vi "RSZVB Get Pulse Train Segments.vi"(8 "error in (no error)":errorcluster {"code" format="%.0x"}, 10 "Channel (1)":i32=1, 11 "VISA session":refnum<visa-resource-name>) -> (0 "error out":errorcluster {"code" format="%.0x"}, 1 "Pulse Train Active":i32[](array[numeric]), 3 "dup VISA session":refnum<visa-resource-name>, 4 "Start Time":dbl[](array[numeric]) format="%^.3e", 5 "Stop Time":dbl[](array[numeric]) format="%^.3e")   [LabVIEW 2011]
doc: "This VI returns the pulse train segments. Each segment consists of a single pulse of definite width and position which may be active or inactive.\n\nNote(s):\n\n(1) This VI is available only with option R&S ZVA-K27.\n\nRemote-control command(s):\n[SENSe<Ch>:]PULSe:GENerator<gen_no>:TRAin:DATA?"
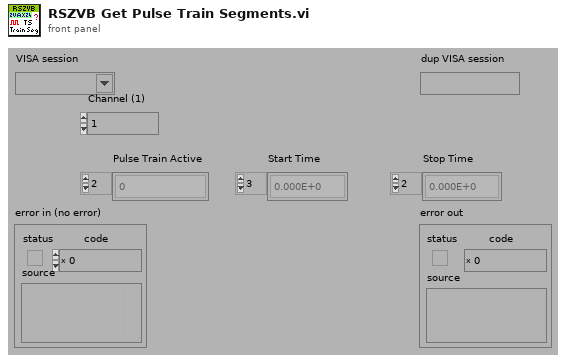
[diagram p1: front panel]
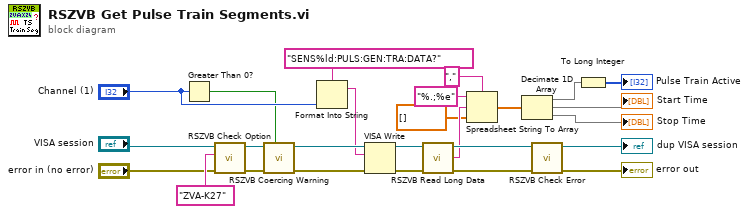
[diagram p0: block diagram]
diagram:
  n1 = Greater Than 0?(x="Channel (1)") -> (x > 0?=w16:bool)
  n2 = call "RSZVB Check Option.vi"("error in (no error)"="error in (no error)", "Options"="ZVA-K27", "VISA session"="VISA session") -> ("error out"=w22:errorcluster, "dup VISA session"=w21:refnum<visa-resource-name>)  [unwired: 7 in]
  n3 = call "RSZVB Coercing Warning.vi"("In Range?"=w16, "error in (no error)"=w22, "VISA session"=w21) -> ("error out"=w25:errorcluster, "dup VISA session"=w26:refnum<visa-resource-name>)  [unwired: 7 in]
  n4 = Format Into String(format string="SENS%ld:PULS:GEN:TRA:DATA?", "Channel (1)") -> (resulting string=w24:string)  [unwired: 2 in, 1 out]
  n5 = VISA Write(VISA resource name=w26, write buffer=w24, error in (no error)=w25) -> (VISA resource name out=w15:refnum<visa-resource-name>, error out=w14:errorcluster)  [unwired: 1 out]
  n6 = call "RSZVB Read Long Data.vi"("error in (no error)"=w14, "VISA resource name"=w15) -> ("error out"=w13:errorcluster, "Data"=w10:string, "VISA resource name out"=w12:refnum<visa-resource-name>)  [unwired: 7 in]
  n7 = Spreadsheet String To Array(delimiter (Tab)=",", format string="%.;%e", spreadsheet string=w10, array type (2D Dbl)=dbl[] [] ("Stop Time")) -> (array=w8:dbl[])
  n8 = Decimate 1D Array(w8) -> (w6:dbl[], →"Start Time":dbl[], →"Stop Time":dbl[])
  n9 = call "RSZVB Check Error.vi"("error in (no error)"=w13, "VISA session"=w12) -> ("error out"=→"error out":errorcluster, "dup VISA session"=→"dup VISA session":refnum<visa-resource-name>)  [unwired: 8 in]
  n10 = To Long Integer(number=w6) -> (32bit integer=→"Pulse Train Active":i32[])
